vi "MeasurementMode.vi"() -> ()   [LabVIEW 2017]
panel:
  in  "VISA resource name":refnum<visa-resource-name>
  out "F-format string":string
  in  "Sampling Interval (min)":dbl format="%.3f"
  in  "Measurement Mode":enum16{"Continuous", "Sample and Hold"}(ring)
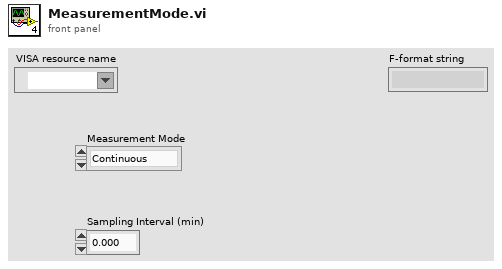
[diagram p1: front panel]
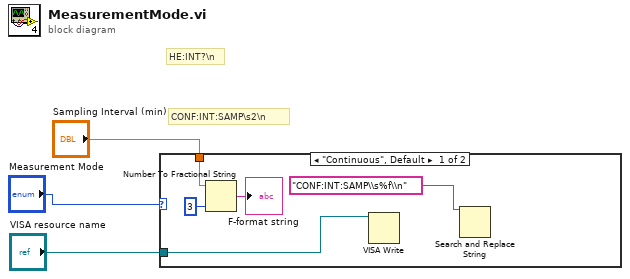
[diagram p0: block diagram]
diagram:
  # "CONF:INT:SAMP\\s2\\n"
  # "HE:INT?\\n"
  n1 = case shown="\"Continuous\", Default" "Measurement Mode" {
    tunnel: "Sampling Interval (min)" -> [w8 _]
    tunnel: "VISA resource name" -> [w5 _]
    frame "Continuous", Default {
      n2 = Number To Fractional String(number=w8, precision (6)=i16 3) -> (F-format string=→"F-format string":string)  [unwired: 2 in]
      n3 = VISA Write(VISA resource name=w5) -> ()  [unwired: 2 in, 3 out]
      n4 = Search and Replace String(input string="CONF:INT:SAMP\\s%f\\n" ("F-format string 2")) -> ()  [unwired: 7 in, 4 out]
    }
    frame "Sample and Hold" {
    }
  }
